vi "Mindsensors Relay Driver.GetTerminals.vi"() -> (1 "Terminals":T1[](array[typedef]) {"Terminal Type" items=["Undefined", "NXT Motor", "NXT Sensor", "HT Daisy Chain", "HT DC Motor", "HT Servo", "HT Touch MUX", "Tetrix Servo", "Tetrix DC Motor", "HT SensorMUX"]})   [LabVIEW 2010]
uses:
  Datatypes/Terminal.ctl
  Datatypes/TerminalType.ctl
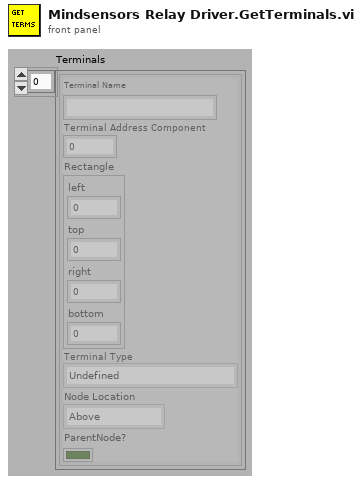
[diagram p1: front panel]
types:
  T1 = typedef "Terminal.ctl" = cluster{"Terminal Name":string, "Terminal Address Component":i16, "Rectangle":cluster{"left":i16, "top":i16, "right":i16, "bottom":i16}, "Terminal Type":T2, "Node Location":enum16{"Above", "Below", "Either"}, "ParentNode?":bool}
  T2 = typedef "TerminalType.ctl" = u16
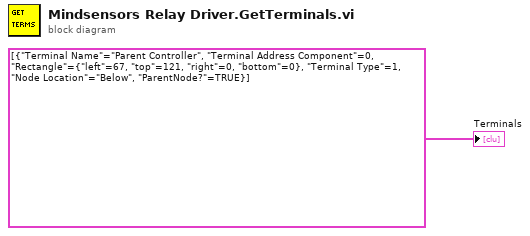
[diagram p0: block diagram]
diagram:
  "Terminals" <- T1[] [{"Terminal Name"="Parent Controller", "Terminal Address Component"=0, "Rectangle"={"left"=67, "top"=121, "right"=0, "bottom"=0}, "Terminal Type"=1, "Node Location"=enum."Below", "ParentNode?"=TRUE}] ("Terminals")
